vi "Probator3000.vi"() -> ()   [LabVIEW 2014]
doc: "Use this template to build a producer/consumer design pattern with events to produce queue items. Use this design pattern instead of the User Interface Event Handler pattern for user interfaces when you want to execute code asynchronously in response to an event without slowing the user interface responsiveness."
uses:
  SELECTOR PRUEBA CAP-USB.ctl
  CAP-USB.lvlib
panel:
  out "Transductores":sgl[](array[numeric])
  out "Valor Encoder":u16
  in  "Num de tramas":i32=200
  out "Raw data":T1(array[cluster])
  out "Waveform Chart":u16(graph)
  in  "INIT":bool
  in  "stop":bool
  in  "VISA resource name":refnum<visa-resource-name>
  in  "error in (no error)":errorcluster
  in  "START-DAQ":bool
  in  "STOP-DAQ":bool
  in  "OPEN-PORT":bool
  in  "CLOSE-PORT":bool
  in  "SALIDAS":bool[](array[boolean])
  out "Entradas":bool[](array[boolean])
  out "Salidas":bool[](array[boolean])
  out "Encoder":dbl(knob)
  in  "DELAY":i32
  in  "TRANSD":bool[](array[boolean])
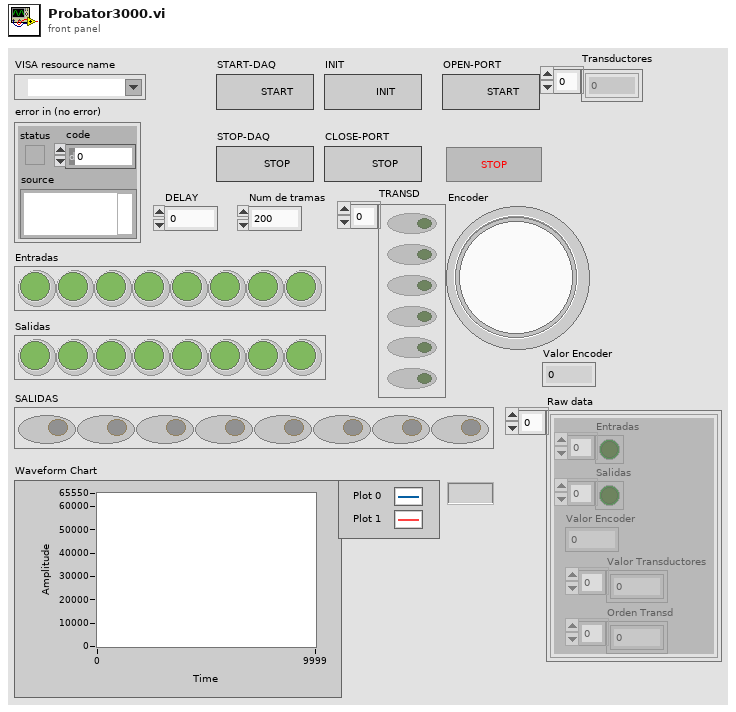
[diagram p1: front panel]
types:
  T1 = cluster{"Entradas":bool[], "Salidas":bool[], "Valor Encoder":u16, "Valor Transductores":u16[], "Orden Transd":i32[]}[]
  T2 = typedef "SELECTOR PRUEBA CAP-USB.ctl" = enum16{"START DAQ", "STOP DAQ", "OPEN PORT", "CLOSE PORT", "STOP", "DAQ", "WRITE PORT", "INIT"}
  T3 = cluster{"Entradas":bool[], "Salidas":bool[], "Valor Encoder":u16, "Valor Transductores":u16[], "Orden Transd":i32[]}
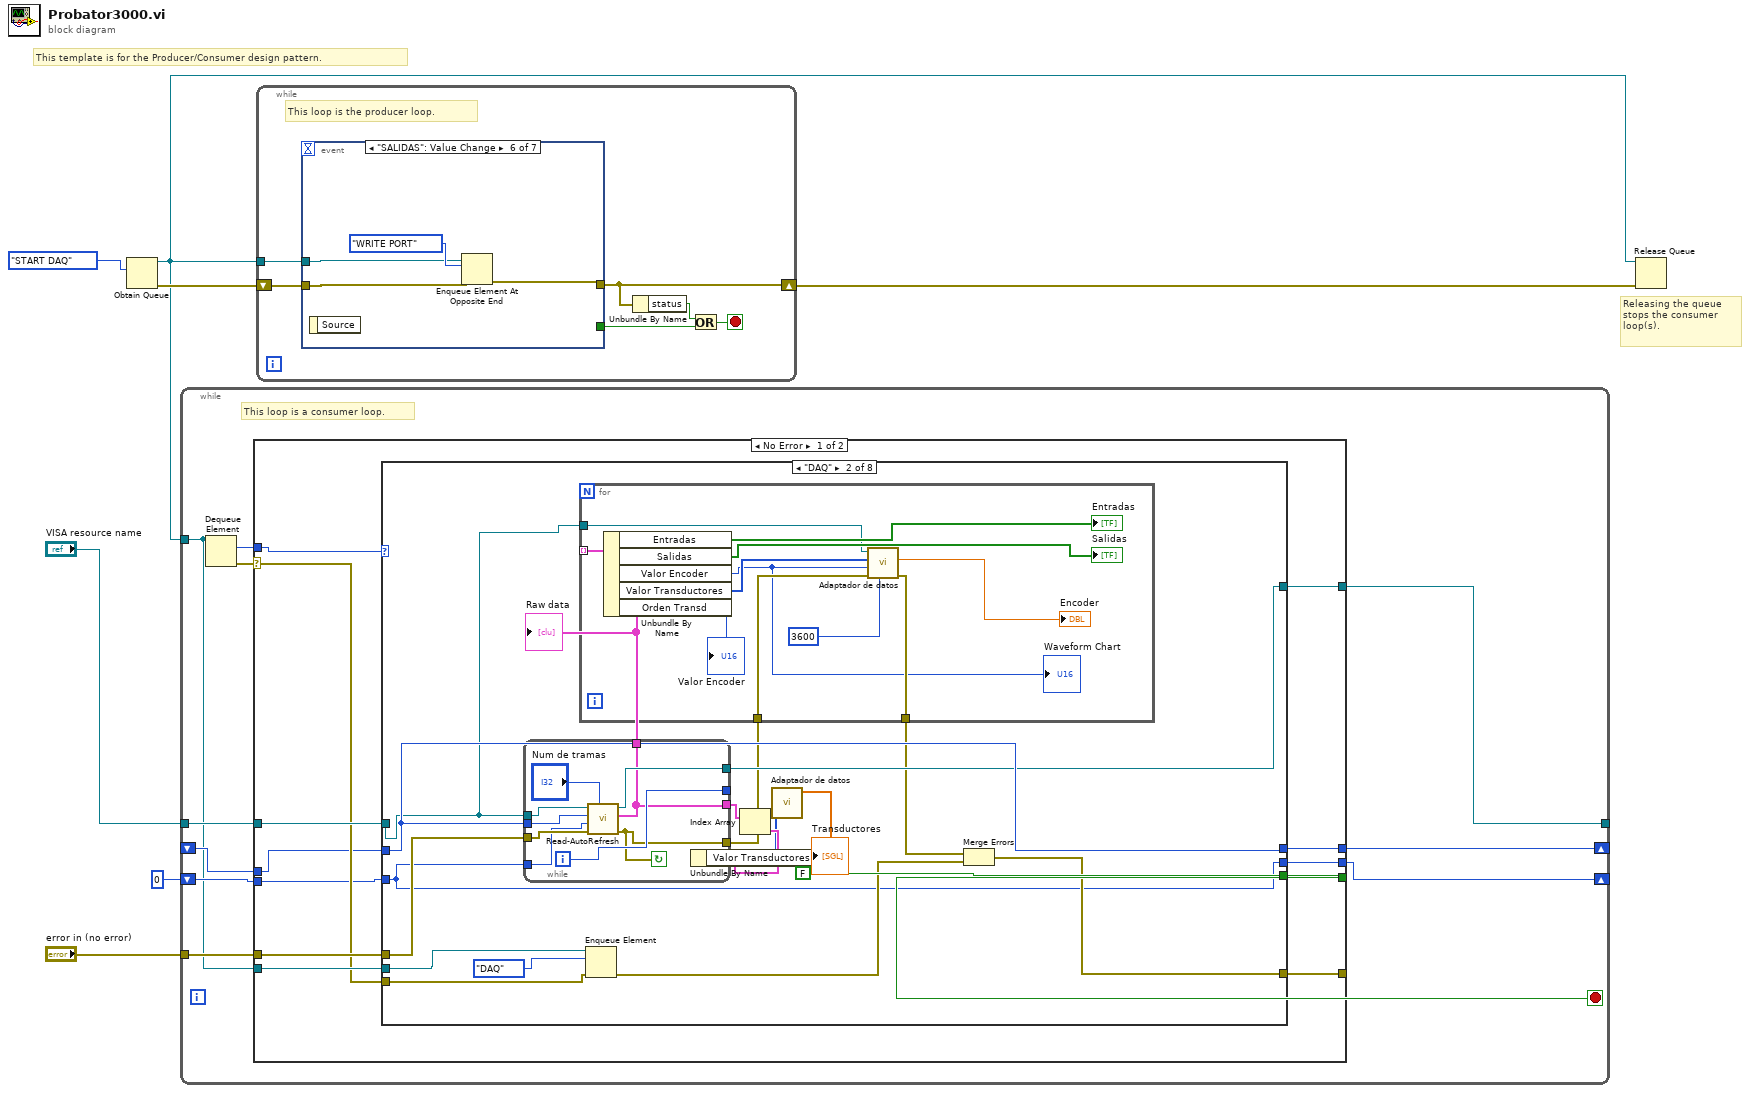
[diagram p0: block diagram]
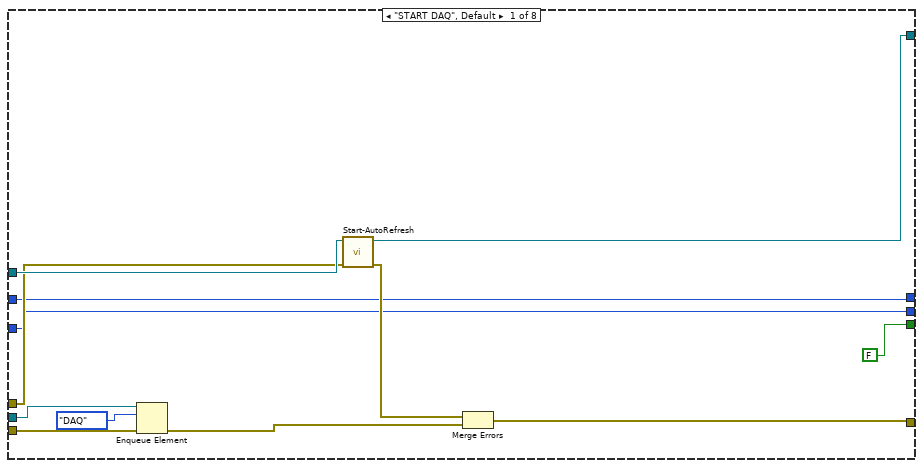
[diagram p2: hidden frame]
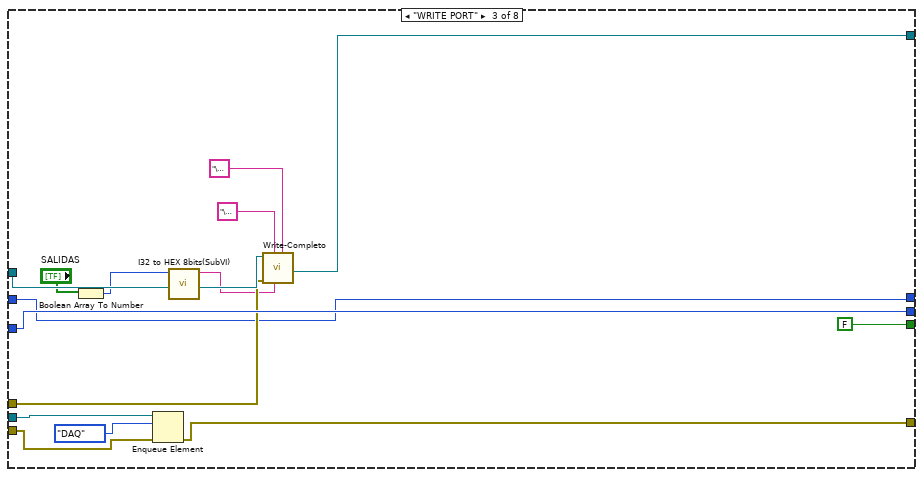
[diagram p3: hidden frame]
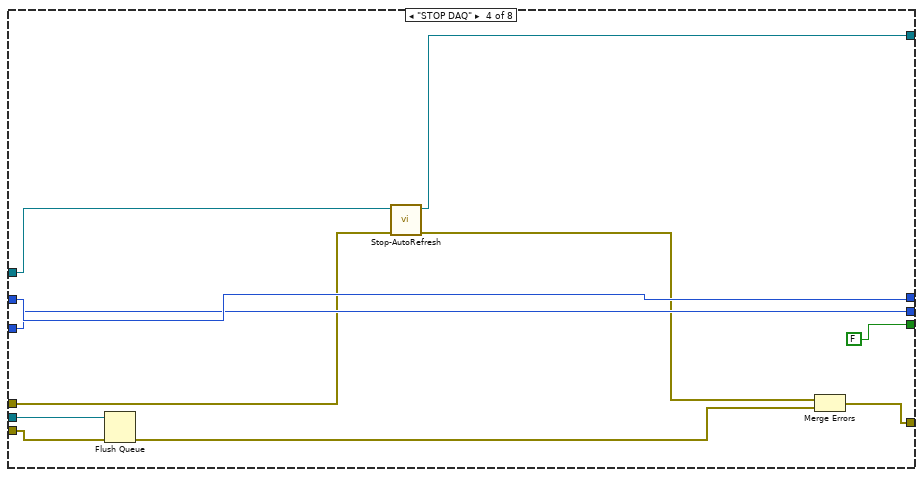
[diagram p4: hidden frame]
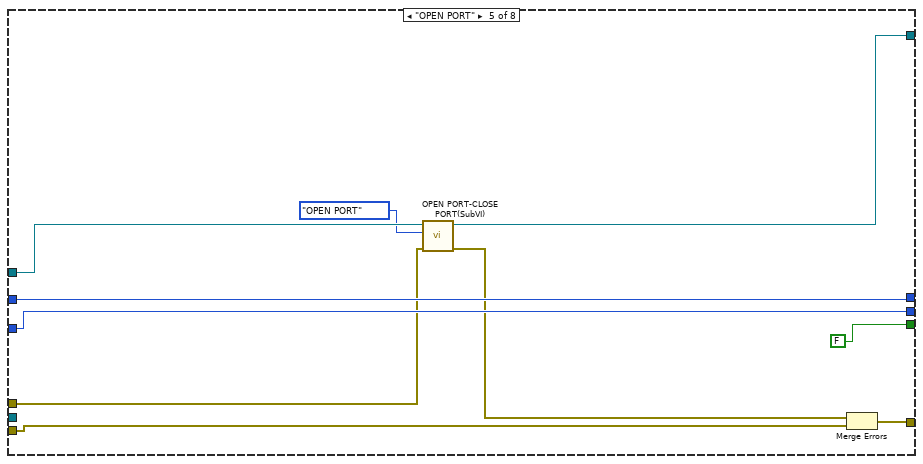
[diagram p5: hidden frame]
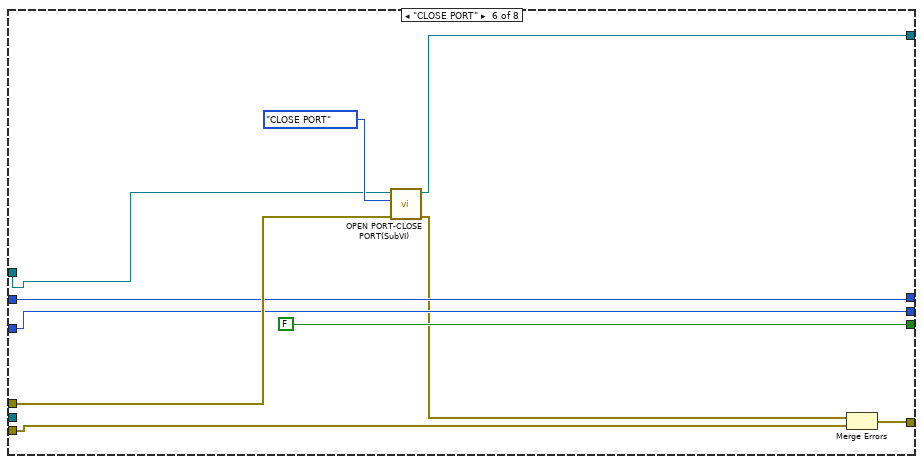
[diagram p6: hidden frame]
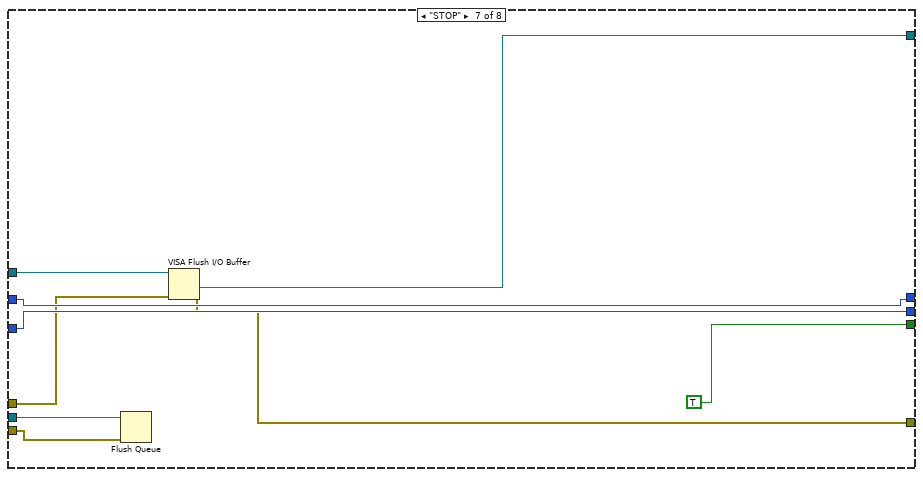
[diagram p7: hidden frame]
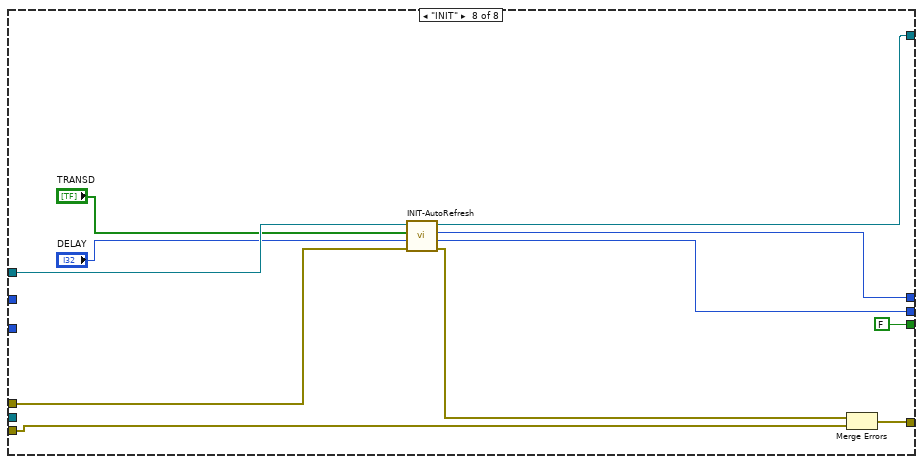
[diagram p8: hidden frame]
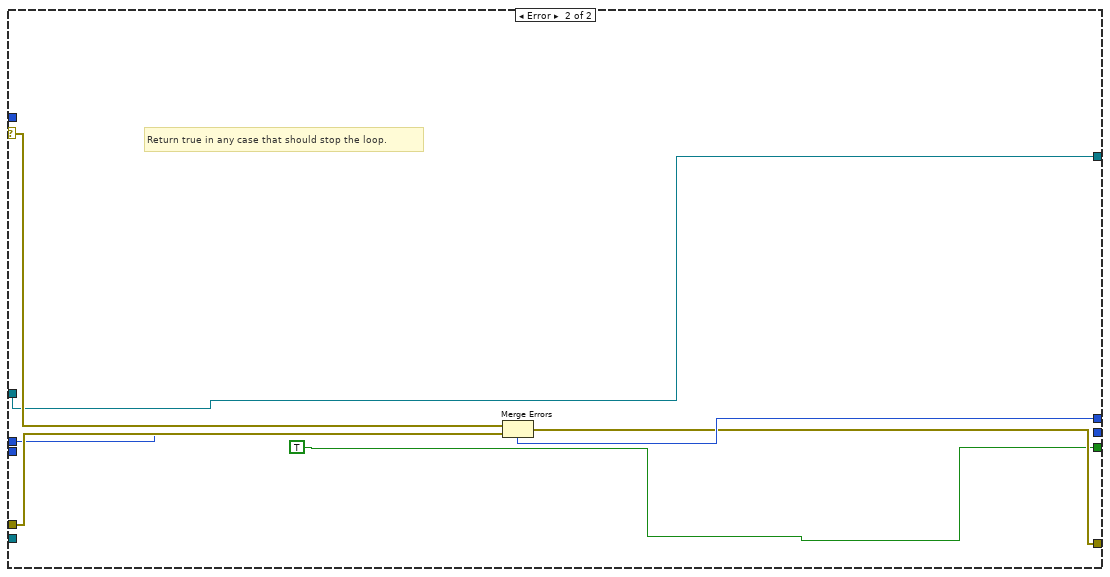
[diagram p9: hidden frame]
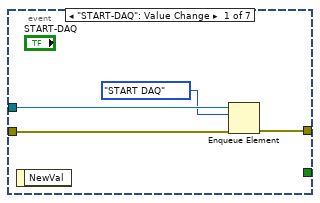
[diagram p10: hidden frame]
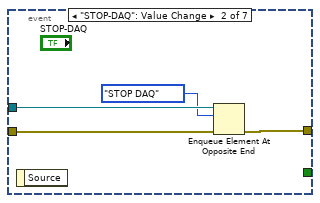
[diagram p11: hidden frame]
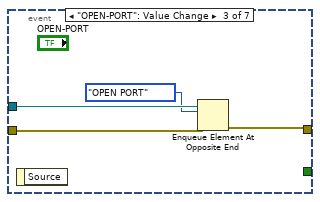
[diagram p12: hidden frame]
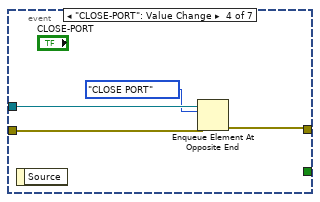
[diagram p13: hidden frame]
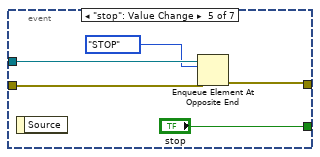
[diagram p14: hidden frame]
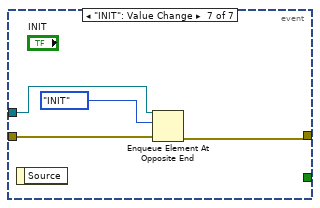
[diagram p15: hidden frame]
diagram:
  # "Releasing the queue stops the consumer loop(s)."
  # "This template is for the Producer/Consumer design pattern."
  n1 = Obtain Queue(element data type=SELECTOR_PRUEBA_CAP-USB."START DAQ") -> (queue out=w5:refnum<queue>, error out=w7:errorcluster)  [unwired: 4 in, 1 out]
  n2 = while {
    tunnel: w5 -> [w8]
    tunnel: "VISA resource name" -> [w15]
    tunnel: "error in (no error)" -> [w14]
    tunnel: [w13] -> _
    shift-right: [w12] -> _
    shift-left: _ -> [w11]
    shift-right: [w10] -> _
    shift-left: 0 ("Tamaño trama") -> [w9]
    stop <- w16 stop-if-true
    # "This loop is a consumer loop."
    n3 = Dequeue Element(queue=w8) -> (element=w17:T2, error out=w18:errorcluster)  [unwired: 2 in, 2 out]
    n4 = case shown="No Error" w18 {
      selector: w18 -> [w24 w151]
      tunnel: w17 -> [w21 _]
      tunnel: [w30 TRUE] -> w16
      tunnel: w15 -> [w29 w149]
      tunnel: w14 -> [w28 w150]
      tunnel: [w27 w149] -> w13
      tunnel: [w26 w147] -> _
      tunnel: w8 -> [w25 _]
      tunnel: [w23 w148] -> w12
      tunnel: w11 -> [w22 w148]
      tunnel: [w20 _] -> w10
      tunnel: w9 -> [w19 _]
      frame No Error {
        n5 = case shown="\"DAQ\"" w21 {
          tunnel: [FALSE FALSE FALSE FALSE FALSE FALSE TRUE FALSE] -> w30
          tunnel: w29 -> [w36 w49 w91 w98 w112 w123 w129 w145]
          tunnel: w28 -> [w35 w55 w90 w97 w111 w122 w128 w144]
          tunnel: [w33 w50 w83 w95 w106 w121 w127 w140] -> w27
          tunnel: [w37 w56 w81 w100 w108 w116 w126 w143] -> w26
          tunnel: w25 -> [w41 w59 w92 w103 _ _ w132 _]
          tunnel: w24 -> [w39 w58 w89 w102 w109 w117 w131 w141]
          tunnel: [w31 w52 w82 w104 w114 w120 w133 w136] -> w23
          tunnel: w22 -> [w31 w52 w82 w104 w114 w120 w133 _]
          tunnel: [w32 w53 w94 w99 w113 w119 w130 w135] -> w20
          tunnel: w19 -> [w32 w53 w94 w99 w113 w119 w130 _]
          frame "START DAQ", Default {
            n6 = Enqueue Element(queue=w41, element=SELECTOR_PRUEBA_CAP-USB."DAQ", error in (no error)=w39) -> (error out=w38:errorcluster)  [unwired: 1 in, 2 out]
            n7 = call "Start-AutoRefresh.vi"("error in (no error)"=w35, "VISA resource name"=w36) -> ("error out"=w34:errorcluster, "VISA resource name out"=w33:refnum<visa-resource-name>)  [unwired: 8 in]
            n8 = Merge Errors(w34, w38) -> (w37:errorcluster)
          }
          frame "DAQ" {
            n9 = while {
              tunnel: w53 -> [w75]
              tunnel: w52 -> [w76]
              tunnel: w55 -> [w77]
              tunnel: w49 -> [w78]
              tunnel: [w79] -> _
              tunnel: [w71] -> w51
              tunnel: [w73] -> w50
              tunnel: [w72] -> w48
              tunnel: [w71] -> w45
              i -> [w79]
              stop <- w72 continue-if-true
              n10 = call "Read-AutoRefresh.vi"("Num de tramas"="Num de tramas", "error in (no error)"=w77, "Tamaño Script"=w75, "TRANSDUCTORES"=w76, "VISA Refnum in"=w78) -> ("error out"=w72:errorcluster, "Raw data"=w71:T1, "VISA reference"=w73:refnum<visa-resource-name>)  [unwired: 4 in]
            }
            "Raw data" <- w51
            n11 = for {
              tunnel: w51 -> [w68] mode=indexing
              tunnel: w49 -> [w67]
              tunnel: w48 -> [w66]
              tunnel: [w65] -> w47
              n12 = Unbundle By Name(w68) -> ("Entradas"=→"Entradas":bool[], "Salidas"=→"Salidas":bool[], "Valor Encoder"=w63:u16, "Valor Transductores"=w64:u16[])  [unwired: 1 out]
              "Waveform Chart" <- w63
              "Valor Encoder" <- w63
              n13 = call "Adaptador de datos.vi"("Cant. de pulsos"=u16 3600, "error in (no error)"=w66, "Encoder"=w63, "Transductores"=w64, "VISA resource name"=w67) -> ("error out"=w65:errorcluster, "Encoder"=→"Encoder":sgl)  [unwired: 4 in, 1 out]
            }
            n14 = Enqueue Element(queue=w59, element=SELECTOR_PRUEBA_CAP-USB."DAQ", error in (no error)=w58) -> (error out=w57:errorcluster)  [unwired: 1 in, 2 out]
            n15 = Index Array(array=w45) -> (element=w44:T3)  [unwired: 1 in]
            n16 = Unbundle By Name(w44) -> ("Valor Transductores"=w43:u16[])
            n17 = call "Adaptador de datos.vi"("Transductores"=w43) -> ("Transductores"=→"Transductores":sgl[])  [unwired: 8 in, 2 out]
            n18 = Merge Errors(w47, w57) -> (w56:errorcluster)
          }
          frame "WRITE PORT" {
            n19 = Boolean Array To Number(Boolean array="SALIDAS") -> (number=w85:u32)
            n20 = Enqueue Element(queue=w92, element=SELECTOR_PRUEBA_CAP-USB."DAQ", error in (no error)=w89) -> (error out=w81:errorcluster)  [unwired: 1 in, 2 out]
            n21 = call "I32 to HEX 8bits(SubVI).vi"("IN U64"=w85) -> ("OUT HEX 8BITS"=w84:string)  [unwired: 10 in]
            n22 = call "Write-Completo.vi"("Low Byte"="\u0001" ("Hi Byte"), "Dato 8 bits"=w84, "Hi Byte"="\u0003", "error in (no error)"=w90, "VISA resource name"=w91) -> ("VISA resource name out"=w83:refnum<visa-resource-name>)  [unwired: 5 in, 1 out]
          }
          frame "STOP DAQ" {
            n23 = Flush Queue(queue=w103, error in (no error)=w102) -> (error out=w101:errorcluster)  [unwired: 2 out]
            n24 = call "Stop-AutoRefresh.vi"("error in (no error)"=w97, "VISA resource name"=w98) -> ("error out"=w96:errorcluster, "VISA resource name out"=w95:refnum<visa-resource-name>)  [unwired: 8 in]
            n25 = Merge Errors(w96, w101) -> (w100:errorcluster)
          }
          frame "OPEN PORT" {
            n26 = call "OPEN PORT-CLOSE PORT(SubVI).vi"("error in (no error)"=w111, "Enum"=enum16{"OPEN PORT", "CLOSE PORT"}."OPEN PORT", "VISA Refnum in"=w112) -> ("error out"=w110:errorcluster, "VISA Refnum out"=w106:refnum<visa-resource-name>)  [unwired: 7 in]
            n27 = Merge Errors(w110, w109) -> (w108:errorcluster)
          }
          frame "CLOSE PORT" {
            n28 = call "OPEN PORT-CLOSE PORT(SubVI).vi"("error in (no error)"=w122, "Enum"=enum16{"OPEN PORT", "CLOSE PORT"}."CLOSE PORT", "VISA Refnum in"=w123) -> ("error out"=w118:errorcluster, "VISA Refnum out"=w121:refnum<visa-resource-name>)  [unwired: 7 in]
            n29 = Merge Errors(w118, w117) -> (w116:errorcluster)
          }
          frame "STOP" {
            n30 = Flush Queue(queue=w132, error in (no error)=w131) -> ()  [unwired: 3 out]
            n31 = VISA Flush I/O Buffer(VISA resource name=w129, error in (no error)=w128) -> (VISA resource name out=w127:refnum<visa-resource-name>, error out=w126:errorcluster)  [unwired: 1 in]
          }
          frame "INIT" {
            n32 = call "INIT-AutoRefresh.vi"("error in (no error)"=w144, "DelayuS"="DELAY", "TDX"="TRANSD", "VISA resource name IN"=w145) -> ("error out"=w142:errorcluster, "Tamaño Script"=w135:i32, "TRANSD"=w136:u16, "VISA resource name OUT"=w140:refnum<visa-resource-name>)  [unwired: 4 in]
            n33 = Merge Errors(w142, w141) -> (w143:errorcluster)
          }
        }
      }
      frame Error {
        # "Return true in any case that should stop the loop."
        n34 = Merge Errors(w151, w150) -> (w147:errorcluster)
      }
    }
  }
  n35 = while {
    shift-right: [w153] -> w6
    shift-left: w7 -> [w156]
    tunnel: w5 -> [w157]
    stop <- w154 stop-if-true
    # "This loop is the producer loop."
    n36 = event shown="[5] \"SALIDAS\": Value Change" {
      selector: _ -> [_ _ _ _ _ _ _]
      dyn-events: _ -> [_ _ _ _ _ _ _]
      timeout: _ -> [_ _ _ _ _ _ _]
      tunnel: w157 -> [w161 w165 w167 w171 w177 w181 w185]
      tunnel: w156 -> [w160 w164 w168 w172 w176 w180 w184]
      tunnel: [w159 w163 w169 w173 w175 w179 w183] -> w153
      tunnel: [_ _ _ _ "stop" _ _] -> w155
      event "START-DAQ": Value Change {
        n37 = event-data() -> ()  [unwired: 1 in, 1 out]
        n38 = Enqueue Element(queue=w161, element=SELECTOR_PRUEBA_CAP-USB."START DAQ", error in (no error)=w160) -> (error out=w159:errorcluster)  [unwired: 1 in, 2 out]
      }
      event "STOP-DAQ": Value Change {
        n39 = event-data() -> ()  [unwired: 1 in, 1 out]
        n40 = Enqueue Element At Opposite End(queue=w165, element=SELECTOR_PRUEBA_CAP-USB."STOP DAQ", error in (no error)=w164) -> (error out=w163:errorcluster)  [unwired: 1 in, 2 out]
      }
      event "OPEN-PORT": Value Change {
        n41 = event-data() -> ()  [unwired: 1 in, 1 out]
        n42 = Enqueue Element At Opposite End(queue=w167, element=SELECTOR_PRUEBA_CAP-USB."OPEN PORT", error in (no error)=w168) -> (error out=w169:errorcluster)  [unwired: 1 in, 2 out]
      }
      event "CLOSE-PORT": Value Change {
        n43 = event-data() -> ()  [unwired: 1 in, 1 out]
        n44 = Enqueue Element At Opposite End(queue=w171, element=SELECTOR_PRUEBA_CAP-USB."CLOSE PORT", error in (no error)=w172) -> (error out=w173:errorcluster)  [unwired: 1 in, 2 out]
      }
      event "stop": Value Change {
        n45 = event-data() -> ()  [unwired: 1 in, 1 out]
        n46 = Enqueue Element At Opposite End(queue=w177, element=SELECTOR_PRUEBA_CAP-USB."STOP", error in (no error)=w176) -> (error out=w175:errorcluster)  [unwired: 1 in, 2 out]
      }
      event "SALIDAS": Value Change {
        n47 = event-data() -> ()  [unwired: 1 in, 1 out]
        n48 = Enqueue Element At Opposite End(queue=w181, element=SELECTOR_PRUEBA_CAP-USB."WRITE PORT", error in (no error)=w180) -> (error out=w179:errorcluster)  [unwired: 1 in, 2 out]
      }
      event "INIT": Value Change {
        n49 = event-data() -> ()  [unwired: 1 in, 1 out]
        n50 = Enqueue Element At Opposite End(queue=w185, element=SELECTOR_PRUEBA_CAP-USB."INIT", error in (no error)=w184) -> (error out=w183:errorcluster)  [unwired: 1 in, 2 out]
      }
    }
    n51 = Unbundle By Name(w153) -> ("status"=w152:bool)
    n52 = Or(x=w152, y=w155) -> (x .or. y?=w154:bool)
  }
  n53 = Release Queue(queue=w5, error in (no error)=w6) -> ()  [unwired: 1 in, 3 out]
